vi "Insert Key Value Pair.vi"   [LabVIEW 2017, in "LVJSON.lvlib" / "JSON Object.lvclass"]
uses:
  JSON Object.lvclass
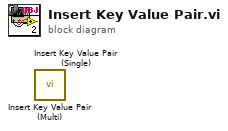
[diagram p0: block diagram]
diagram:
  n1 = call "Insert Key Value Pair (Multi).vi"() -> ()  [unwired: 10 in, 2 out]
  n2 = call "Insert Key Value Pair (Single).vi"() -> ()  [unwired: 10 in, 2 out]
